vi "Unregister Messages.vi"(8 "error in (no error)":errorcluster, 10 "Message Unregistration":T1, 11 "Remote Messaging Module in":refnum<class "Remote Messaging Module.lvclass">) -> (0 "error out":errorcluster, 3 "Remote Messaging Module out":refnum<class "Remote Messaging Module.lvclass">)   [LabVIEW 2020, in "Volatus.lvlib" / "Remote Messaging Module.lvclass"]
uses:
  Remote Messaging Module.lvclass
  Message Unregistration.ctl
  MessageQ/MessageQ.lvclass
  Remote Messaging Module.lvclass/Remote Messaging Module.ctl
  Volatus.lvlib
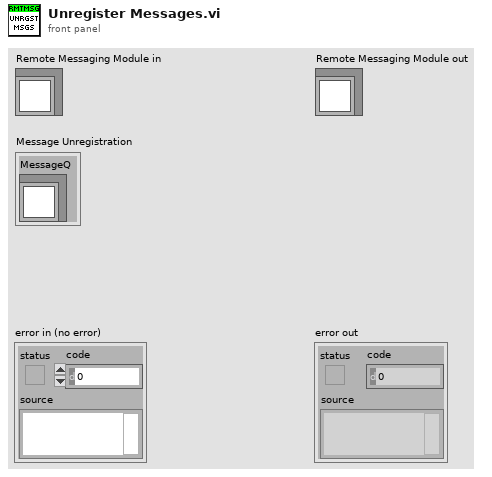
[diagram p1: front panel]
types:
  T1 = typedef "Volatus.lvlib/Message Unregistration.ctl" = cluster{"MessageQ":refnum<class "MessageQ.lvclass">}
  T2 = typedef "Volatus.lvlib/Remote Messaging Module.lvclass/Type Handler.ctl" = cluster{"Msg ID":string, "MsgQ":refnum<class "MessageQ.lvclass">}
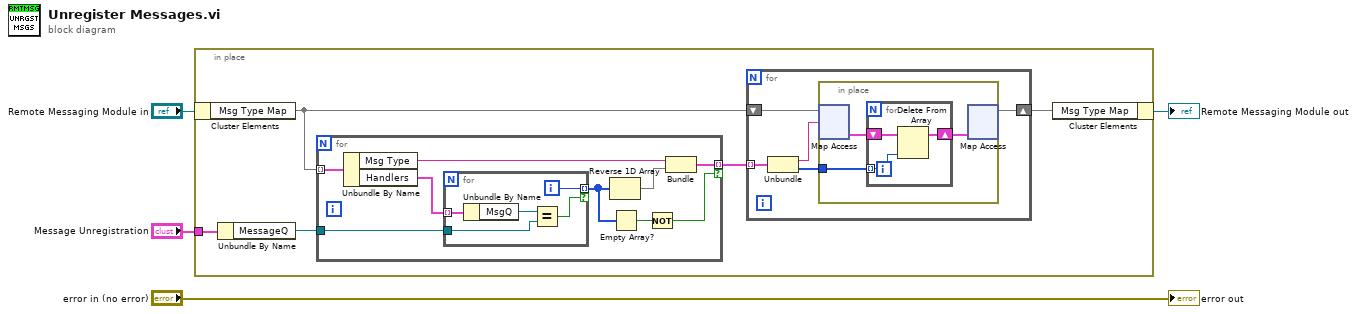
[diagram p0: block diagram]
diagram:
  n1 = in-place {
    in-place-border: "Message Unregistration" -> [w9]
    n2 = in-place-cluster #1("Remote Messaging Module in") -> ("Msg Type Map"=w7:map{string, T2[]})
    n3 = Unbundle By Name(w9) -> ("MessageQ"=w8:refnum<class "MessageQ.lvclass">)
    n4 = for {
      tunnel: w8 -> [w27]
      tunnel: w7 -> [w29] mode=indexing
      tunnel: [w22] -> w6 mode=indexing if=w21
      n5 = Unbundle By Name(w29) -> ("Msg Type"=w25:string, "Handlers"=w28:T2[])
      n6 = for {
        tunnel: w28 -> [w34] mode=indexing
        tunnel: w27 -> [w32]
        tunnel: [w31] -> w26 mode=indexing if=w30
        i -> [w31]
        n7 = Unbundle By Name(w34) -> ("MsgQ"=w33:refnum<class "MessageQ.lvclass">)
        n8 = Equal?(x=w33, y=w32) -> (x = y?=w30:bool)
      }
      n9 = Reverse 1D Array(array=w26) -> (reversed array=w23:i32[])
      n10 = Empty Array?(array=w26) -> (empty?=w24:bool)
      n11 = Not(x=w24) -> (.not. x?=w21:bool)
      n12 = Bundle("Msg Type"=w25, w23) -> (w22:cluster{"Msg Type":string, i32[]})  [unwired: 1 in]
    }
    n13 = for {
      shift-right: [w10] -> w5
      shift-left: w7 -> [w13]
      tunnel: w6 -> [w14] mode=indexing
      n14 = Unbundle(w14) -> ("Msg Type"=w12:string, w11:i32[])
      n15 = in-place {
        in-place-border: w11 -> [w16]
        n16 = in-place-map #2(w13, w12) -> (w17:T2[])  [unwired: 1 in, 1 out]
        n17 = for {
          shift-right: [w18] -> w15
          shift-left: w17 -> [w20]
          tunnel: w16 -> [w19] mode=indexing
          n18 = Delete From Array(array=w20, index=w19) -> (array with subset deleted=w18:T2[])  [unwired: 1 in, 1 out]
        }
        n19 = in-place-map #2(w15) -> (w10:map{string, T2[]})  [unwired: 1 in, 2 out]
      }
    }
    n20 = in-place-cluster #1("Msg Type Map"=w5) -> (→"Remote Messaging Module out":refnum<class "Remote Messaging Module.lvclass">)
  }
  "error out" <- "error in (no error)"
